vi "Init.vi"(5 "Height (Source)":i32, 6 "Quality (90)":i32=90, 7 "Width (Source)":i32, 8 "error in (no error)":errorcluster, 10 "Image Format":string, 11 "Source Name":string) -> (0 "error out":errorcluster, 3 "GetSourceScreenshot out":refnum<class "GetSourceScreenshot.lvclass">)   [LabVIEW 2020, in "obs-websocket.lvlib" / "GetSourceScreenshot.lvclass"]
uses:
  GetSourceScreenshot.lvclass
  GetSourceScreenshot.lvclass/GetSourceScreenshot.ctl
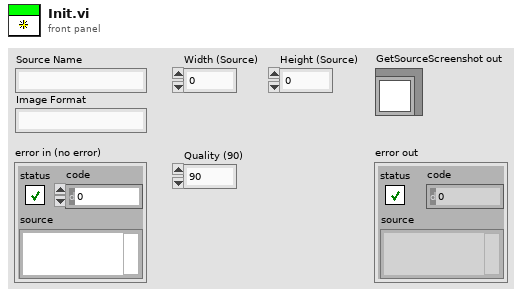
[diagram p1: front panel]
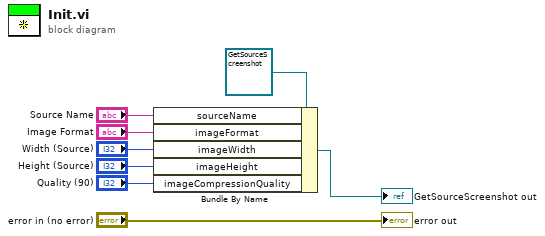
[diagram p0: block diagram]
diagram:
  n1 = Bundle By Name(cluster=refnum<class "GetSourceScreenshot.lvclass"> refnum ("GetSourceScreenshot in"), "sourceName"="Source Name", "imageFormat"="Image Format", "imageWidth"="Width (Source)", "imageHeight"="Height (Source)", "imageCompressionQuality"="Quality (90)") -> (→"GetSourceScreenshot out":refnum<class "GetSourceScreenshot.lvclass">)
  "error out" <- "error in (no error)"
